vi "append_to_log.vi"(5 "data_type":T1, 7 "dims":T2, 8 "error in (no error)":errorcluster, 9 "Location":string, 10 "Data":variant, 11 "data_logger in":refnum<class "data_logger.lvclass">) -> (0 "error out":errorcluster, 3 "data_logger out":refnum<class "data_logger.lvclass">)   [LabVIEW 2015, in "data_logger.lvclass"]
uses:
  data_logger.lvclass
  data_dimensionality.ctl
  logger_data_types.ctl
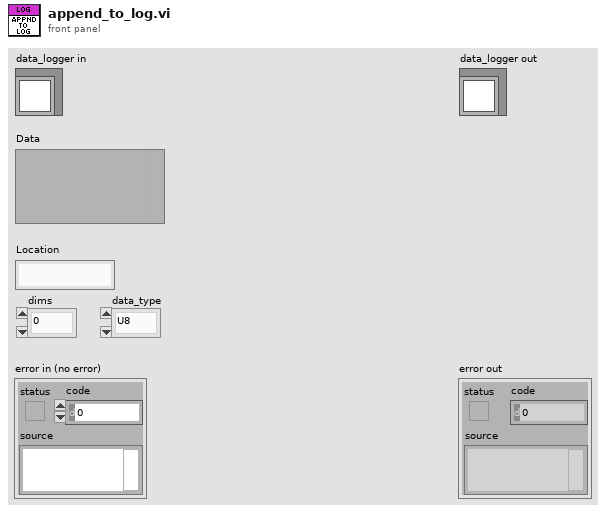
[diagram p1: front panel]
types:
  T1 = typedef "logger_data_types.ctl" = enum16{"U8", "I8", "U16", "I16", "U32", "I32", "DBL", "String"}
  T2 = typedef "data_dimensionality.ctl" = enum16{"0", "1", "2"}
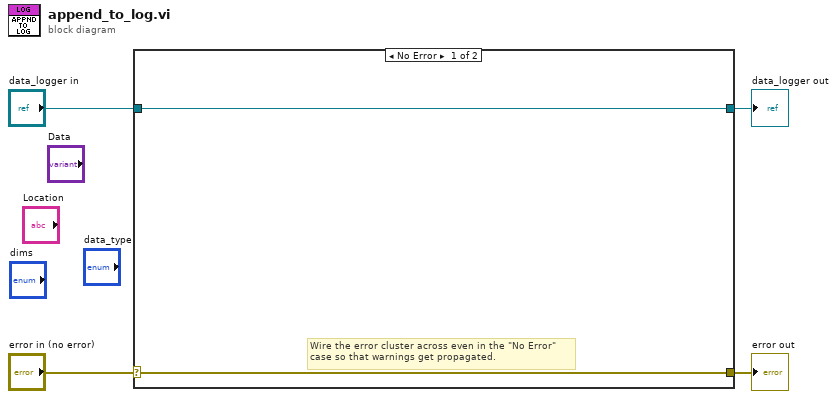
[diagram p0: block diagram]
diagram:
  n1 = case shown="No Error" "error in (no error)" {
    selector: "error in (no error)" -> [w5 w8]
    tunnel: [w5 w8] -> w3
    tunnel: [w6 w7] -> w1
    tunnel: "data_logger in" -> [w6 w7]
    frame No Error {
      # "Wire the error cluster across even in the \"No Error\"\ncase so that warnings get propagated."
    }
    frame Error {
    }
  }
  "error out" <- w3
  "data_logger out" <- w1
